vi "find variables  names by reg exp.vi"(10 "exclude string (reg exp)":string, 11 "search string (reg exp)":string) -> (2 "Array of Variable Names":string[](array[string]), 3 "CRLF delimited string of Variable Names":string)   [LabVIEW 2017]
doc: "SciScan 1.2 160622"
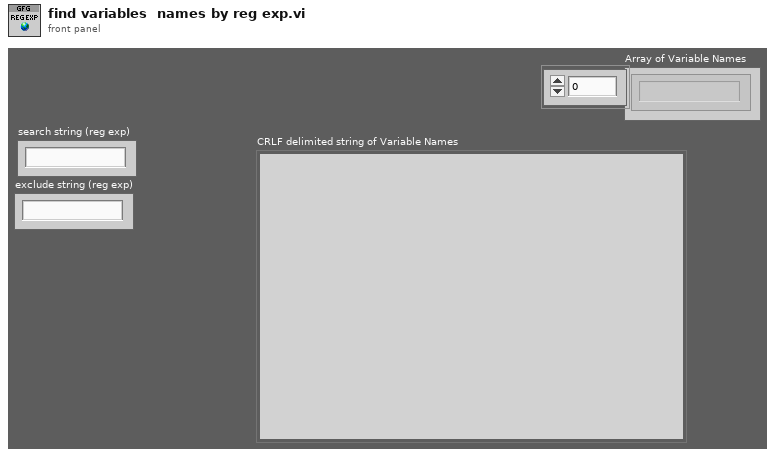
[diagram p1: front panel]
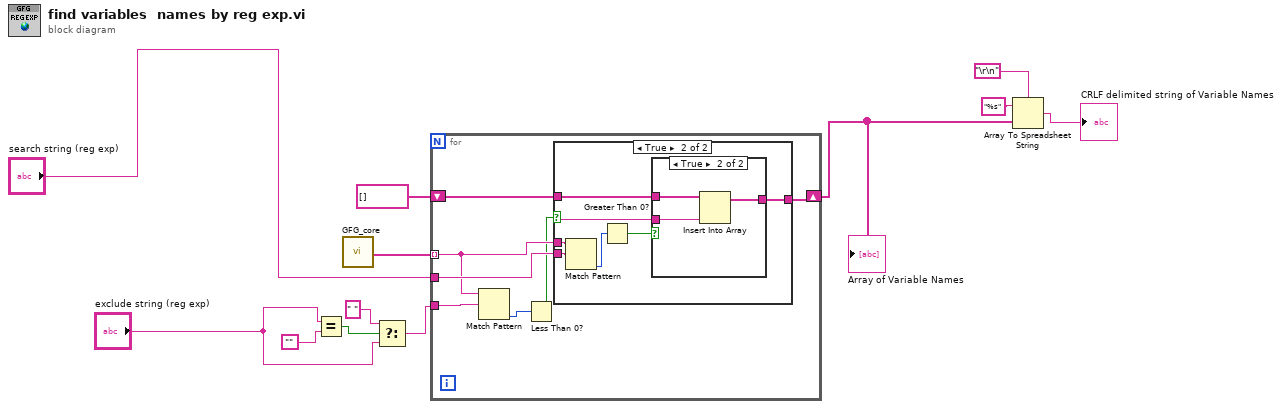
[diagram p0: block diagram]
diagram:
  n1 = Equal?(x="exclude string (reg exp)", y="") -> (x = y?=w5:bool)
  n2 = call "GFG_core.vi"() -> ("All Variable Names Out"=w12:string[])  [unwired: 13 in, 6 out]
  n3 = Select(t=" ", s=w5, f="exclude string (reg exp)") -> (s? t:f=w2:string)
  n4 = for {
    tunnel: w12 -> [w15] mode=indexing
    shift-right: [w18] -> w8
    shift-left: string[] [] ("All Variable Names Out") -> [w19]
    tunnel: "search string (reg exp)" -> [w17]
    tunnel: w2 -> [w16]
    n5 = Match Pattern(string=w15, regular expression=w16) -> (offset past match=w14:i32)  [unwired: 1 in, 3 out]
    n6 = Less Than 0?(x=w14) -> (x < 0?=w13:bool)
    n7 = case shown="True" w13 {
      tunnel: w19 -> [w20 w25]
      tunnel: [w20 w24] -> w18
      tunnel: w17 -> [_ w22]
      tunnel: w15 -> [_ w21]
      frame False {
      }
      frame True {
        n8 = Match Pattern(string=w21, regular expression=w22) -> (offset past match=w26:i32)  [unwired: 1 in, 3 out]
        n9 = Greater Than 0?(x=w26) -> (x > 0?=w23:bool)
        n10 = case shown="True" w23 {
          tunnel: w25 -> [w27 w30]
          tunnel: [w27 w29] -> w24
          tunnel: w21 -> [_ w28]
          frame False {
          }
          frame True {
            n11 = Insert Into Array(array=w30, new element=w28) -> (w29:string[])  [unwired: 1 in]
          }
        }
      }
    }
  }
  "Array of Variable Names" <- w8
  n12 = Array To Spreadsheet String(delimiter (Tab)="\r\n", array=w8, 3:"%s" ("format string")) -> (spreadsheet string=→"CRLF delimited string of Variable Names":string)
